vi "SearchEachElFrom1DToEveryIdxIn2D.vi"(8 "Array":u64[](array[numeric])) -> (0 "Map matching":map{string, i32}(c390), 3 "Matching array":u64[](array[numeric]), 11 "2D Target Array":i32[][](array[numeric]))   [LabVIEW 2023]
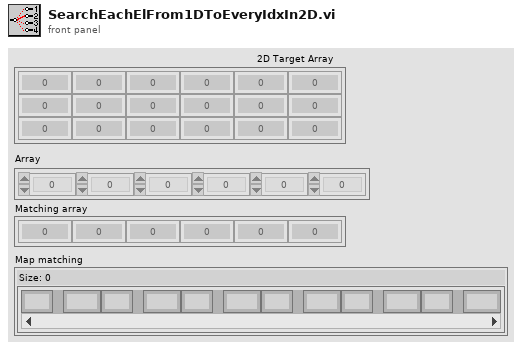
[diagram p1: front panel]
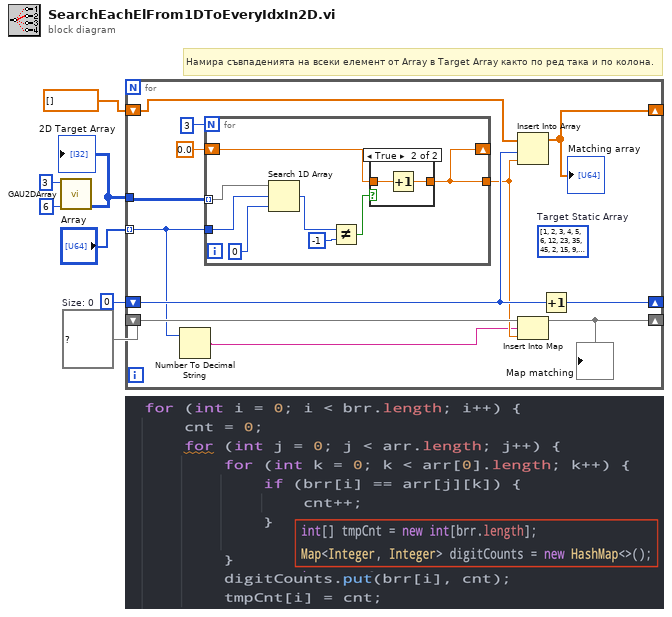
[diagram p0: block diagram]
diagram:
  w1 = map{string, i32} {}  # Size: 0
  # "Намира съвпаденията на всеки елемент от Array в Target Array както по ред така и по колона."
  n1 = call "GAU2DArray.vi"("Colums"=6, "Rows"=3) -> ("2D Double Array"=w2:i32[][])  [unwired: 8 in, 1 out]
  "2D Target Array" <- w2
  n2 = for {
    tunnel: "Array" -> [w9] mode=indexing
    tunnel: w2 -> [w19]
    shift-right: [w16] -> _
    shift-left: dbl[] [] -> [w15]
    shift-right: [w14] -> _
    shift-left: u64 0 -> [w13]
    shift-right: [w12] -> _
    shift-left: w1 -> [w11]
    (unwired) u64[][] [[1, 2, 3, 4, 5, 6], [12, 23, 35, 45, 2, 15], [9, 3, 14, 5, 6, 7]]  # Target Static Array
    n3 = Number To Decimal String(number=w9) -> (decimal integer string=w8:string)  [unwired: 1 in]
    n4 = for {
      N: 3 -> [_]
      tunnel: w19 -> [w27] mode=indexing
      tunnel: w9 -> [w26]
      shift-right: [w20] -> _
      shift-left: 0.0 -> [w22]
      tunnel: [w20] -> w10
      n5 = Search 1D Array(1D array=w27, element=w26, start index (0)=0) -> (index of element=w25:i32)
      n6 = Not Equal?(x=w25, y=-1) -> (x != y?=w23:bool)
      n7 = case shown="True" w23 {
        tunnel: [w28 w30] -> w20
        tunnel: w22 -> [w28 w29]
        frame False {
        }
        frame True {
          n8 = Increment(x=w29) -> (x+1=w30:dbl)
        }
      }
    }
    n9 = Insert Into Array "Insert Into Array"(array=w15, index=w13, new element=w10) -> (w16:dbl[])
    "Matching array" <- w16
    n10 = Insert Into Map(map in=w11, key=w8, value=w10) -> (map out=w12:map{string, i32})  [unwired: 2 out]
    "Map matching" <- w12
    n11 = Increment(x=w13) -> (x+1=w14:u64)
  }
